vi "Backup LabVIEW.ini File.vi"(8 "error in (no error)":errorcluster) -> (0 "error out":errorcluster, 3 "new path":path)   [LabVIEW 2012]
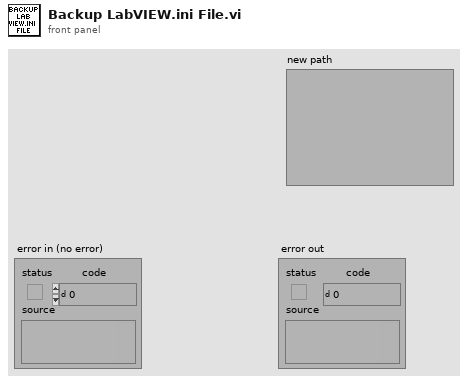
[diagram p1: front panel]
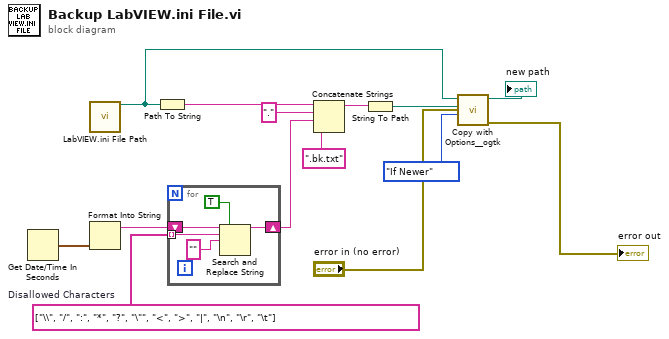
[diagram p0: block diagram]
diagram:
  w3 = string[] ["\\", "/", ":", "*", "?", "\"", "<", ">", "|", "\n", "\r", "\t"]  # Disallowed Characters
  n1 = Get Date/Time In Seconds() -> (seconds since 1Jan1904=w5:timestamp)
  n2 = call "LabVIEW.ini File Path.vi"() -> ("appended path"=w11:path)  [unwired: 19 in]
  n3 = Format Into String(w5) -> (resulting string=w2:string)  [unwired: 3 in, 1 out]
  n4 = Path To String(path=w11) -> (string=w14:string)
  n5 = for {
    tunnel: w3 -> [w17] mode=indexing
    shift-right: [w15] -> w1
    shift-left: w2 -> [w18]
    n6 = Search and Replace String(replace all?=TRUE ("replace all? (F)"), input string=w18, search string=w17, replace string="" ("replace string (\"\")")) -> (result string=w15:string)  [unwired: 4 in, 3 out]
  }
  n7 = Concatenate Strings(w14, "." ("string"), w1, ".bk.txt" ("string")) -> (w12:string)
  n8 = String To Path(string=w12) -> (path=w10:path)
  n9 = call <userlib>:"Copy with Options__ogtk.vi"("error in (no error)"="error in (no error)", "Replace Mode (Never)"=enum16{"Never", "Always", "If Newer"}."If Newer", "target path"=w10, "source path"=w11) -> ("error out"=→"error out":errorcluster, "new path"=→"new path":path)  [unwired: 6 in]
